vi "myRIO_BRig_RT_dataMTrig_CueLed_c.vi"() -> (2 "output_CueLed_c":i32)   [LabVIEW 2014]
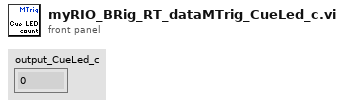
[diagram p1: front panel]
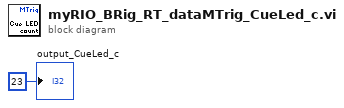
[diagram p0: block diagram]
diagram:
  "output_CueLed_c" <- 23 ("output_iBlock")
